vi "Purge PH - API.vi"(6 "Timeout (ms)":u32=5000, 7 "Wait (F)":bool, 8 "error in (no error)":errorcluster, 9 "Duration (s)":dbl, 10 "ICP1-DO Channel Name":T1, 11 "IO in":refnum<class "IO.lvclass">) -> (0 "error out":errorcluster, 3 "IO out":refnum<class "IO.lvclass">)   [LabVIEW 2022 SP3, in "IO.lvclass"]
uses:
  IO.lvclass
  Typedefs/ICP1-D0 Channel Names.ctl
  Typedefs/API Command Cluster.ctl
  Typedefs/API Command Enum.ctl
  Typedefs/Purge PH API Data.ctl
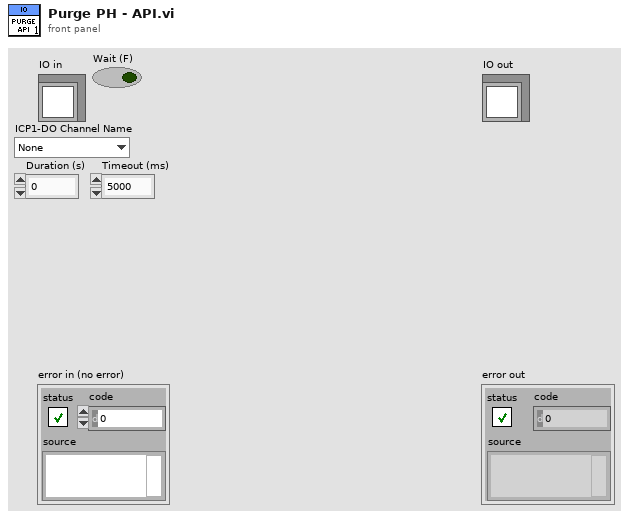
[diagram p1: front panel]
types:
  T1 = typedef "IO.lvclass/ICP1-D0 Channel Names.ctl" = enum16{"None", "Meniscus Pressure Reg PWR - R1", "Meniscus Pressure Reg PWR - R2", "Meniscus Pressure Reg PWR - R3", "Meniscus Pressure Reg PWR - R4", "Meniscus Pressure Reg PWR - R5", "Meniscus Pressure Reg PWR - R6", "Clear Stage Alarm", "Servo ON", "Purge Valve Open - R1", "Purge Valve Open - R2", "Purge Valve Open - R3", "Purge Valve Open - R4", "Purge Valve Open - R5", "Purge Valve Open - R6"}
  T2 = typedef "IO.lvclass/Purge PH API Data.ctl" = cluster{"ICP1-DO Channel Name":T1, "Duration (s)":dbl}
  T3 = typedef "IO.lvclass/API Command Enum.ctl" = enum16{"Set DO Value", "Set AO Value", "Purge PH"}
  T4 = typedef "IO.lvclass/API Command Cluster.ctl" = cluster{"Command":T3, "Arguments":string, "Data":variant}
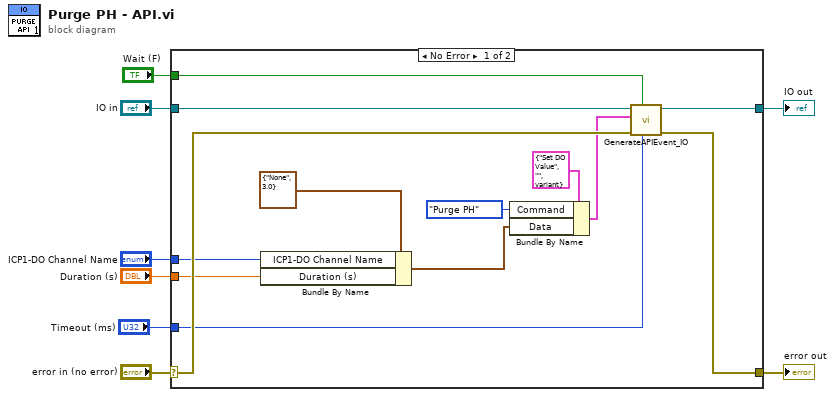
[diagram p0: block diagram]
diagram:
  n1 = case shown="No Error" "error in (no error)" {
    selector: "error in (no error)" -> [w20 w23]
    tunnel: [w19 w23] -> w7
    tunnel: [w21 w22] -> w5
    tunnel: "IO in" -> [w11 w22]
    tunnel: "Duration (s)" -> [w13 _]
    tunnel: "ICP1-DO Channel Name" -> [w12 _]
    tunnel: "Wait (F)" -> [w10 _]
    tunnel: "Timeout (ms)" -> [w9 _]
    frame No Error {
      n2 = Bundle By Name(cluster=T2 {"ICP1-DO Channel Name"=enum."None", "Duration (s)"=3.0} ("Purge PH API Data"), "ICP1-DO Channel Name"=w12, "Duration (s)"=w13) -> (w14:T2)
      n3 = Bundle By Name(cluster=T4 {"Command"=enum."Set DO Value", "Arguments"="", "Data"=variant} ("API Command Cluster"), "Command"=API_Command_Enum."Purge PH", "Data"=w14) -> (w16:T4)
      n4 = call "GenerateAPIEvent_IO.vi"("Timeout (ms)"=w9, "Wait (F)"=w10, "error in (no error)"=w20, "API Command Cluster"=w16, "IO.lvclass"=w11) -> ("error out"=w19:errorcluster, "IO.lvclass out"=w21:refnum<class "IO.lvclass">)  [unwired: 5 in]
    }
    frame Error {
    }
  }
  "error out" <- w7
  "IO out" <- w5
